vi "Test Process Log Handler Configured.vi"(8 "error in (no error)":errorcluster, 11 "Process Test In":refnum<class "Process Test.lvclass">) -> (0 "error out":errorcluster, 3 "Process Test Out":refnum<class "Process Test.lvclass">)   [LabVIEW 2020, in "Process Test.lvclass"]
uses:
  Process Test.lvclass
  C:/Program Files (x86)/National Instruments/LabVIEW 2020/vi.lib/Asteme/LUnit/Test Case.lvclass
  Mock Log Handler/Mock Log Handler.lvclass
  C:/Users/anton/Documents/GitHub/Triarc-Framework/source/Framework/Logging/Logging.lvclass
  <vilib>/Asteme/LUnit/Test Case.lvclass/Test Case.ctl
  <vilib>/Asteme/LUnit/LUnit Assertion Result.lvclass/LUnit Assertion Result.ctl
  <vilib>/Asteme/LUnit/Palette/Pass If.vi
  <vilib>/Asteme/LUnit/Set Assertion Type.vi
  <vilib>/Asteme/LUnit/Palette/Fail.vi
  <vilib>/Asteme/LUnit/Palette/Pass.vi
  <vilib>/Asteme/LUnit/LUnit Write Assertion Type.vi
  <vilib>/Asteme/LUnit/Add test result.vi
  <vilib>/Asteme/LUnit/LUnit Write Passed.vi
  <vilib>/Asteme/LUnit/LUnit Get Test Case.vi
  <vilib>/Asteme/LUnit/Assertion Result/LUnit Get Test Name.vi
  <vilib>/Asteme/LUnit/LUnit Write Message.vi
  <vilib>/Asteme/LUnit/LUnit Write Description.vi
  <vilib>/Asteme/LUnit/Read Test Case Name.vi
  <vilib>/Asteme/LUnit/LUnit Assertion Result.lvclass
  Framework/Process/Process.lvclass
  <vilib>/Asteme/LUnit/Test Case.lvclass
  C:/Users/anton/Documents/GitHub/Triarc-Framework/source/Framework/Base/Base.lvclass
  C:/Users/anton/Documents/GitHub/Triarc-Framework/source/Framework Test/Mock Log Handler/Mock Log Handler.lvclass
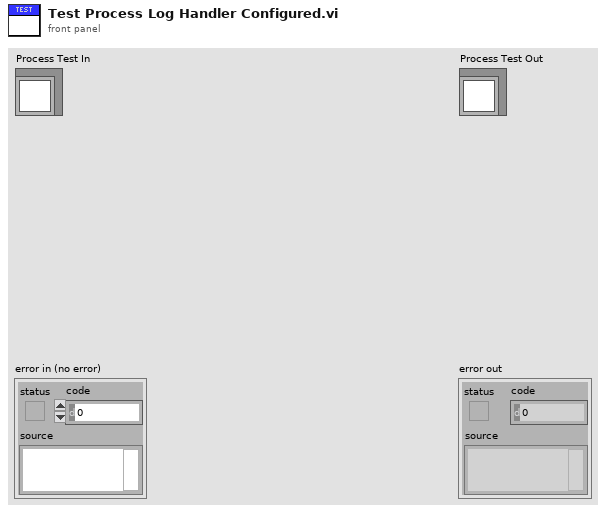
[diagram p1: front panel]
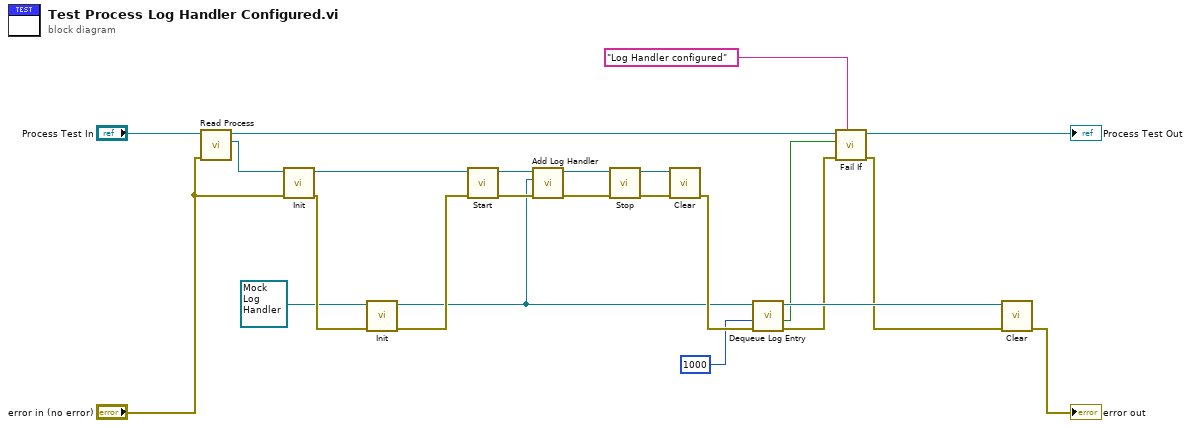
[diagram p0: block diagram]
diagram:
  n1 = call "Read Process.vi"("error in (no error)"="error in (no error)", "Process Test in"="Process Test In") -> ("Process.lvclass"=w12:refnum<class "Process.lvclass">, "Process Test out"=w11:refnum<class "Process Test.lvclass">)  [unwired: 7 in, 1 out]
  n2 = call-dynamic "Init.vi"("error in (no error)"="error in (no error)", "Process In"=w12) -> ("error out"=w23:errorcluster, "Process Out"=w3:refnum<class "Process.lvclass">)  [unwired: 8 in]
  n3 = call-dynamic "Init.vi"("error in (no error)"=w23, "Mock Log Handler In"=refnum<class "Mock Log Handler.lvclass"> refnum ("Mock Log Handler.lvclass")) -> ("error out"=w19:errorcluster, "Mock Log Handler Out"=w1:refnum<class "Mock Log Handler.lvclass">)  [unwired: 8 in]
  n4 = call "Start.vi"("error in (no error)"=w19, "Process In"=w3) -> ("error out"=w4:errorcluster, "Process Out"=w2:refnum<class "Process.lvclass">)  [unwired: 8 in]
  n5 = call "Add Log Handler.vi"("error in (no error)"=w4, "Log Handler"=w1, "Process In"=w2) -> ("error out"=w20:errorcluster, "Process Out"=w21:refnum<class "Process.lvclass">)  [unwired: 7 in]
  n6 = call "Stop.vi"("error in (no error)"=w20, "Process In"=w21) -> ("error out"=w6:errorcluster, "Process Out"=w5:refnum<class "Process.lvclass">)  [unwired: 7 in, 1 out]
  n7 = call-dynamic "Clear.vi"("error in (no error)"=w6, "Process In"=w5) -> ("error out"=w16:errorcluster)  [unwired: 9 in]
  n8 = call "Dequeue Log Entry.vi"("error in (no error)"=w16, "timeout in ms (-1)"=1000, "Mock Log Handler in"=w1) -> ("error out"=w15:errorcluster, "timed out?"=w7:bool, "Mock Log Handler out"=w18:refnum<class "Mock Log Handler.lvclass">)  [unwired: 5 in, 1 out]
  n9 = call <vilib>:"Fail If.vi"("Description"="Log Handler configured", "error in (no error)"=w15, "Fail?"=w7, "Test Case In"=w11) -> ("error out"=w14:errorcluster, "Test Case Out"=→"Process Test Out":refnum<class "Process Test.lvclass">)  [unwired: 6 in]
  n10 = call-dynamic "Clear.vi"("error in (no error)"=w14, "Mock Log Handler In"=w18) -> ("error out"=→"error out":errorcluster)  [unwired: 9 in]
